vi "VI Anlagenuebersicht PNS.vi"() -> (3 "XML-String":string)   [LabVIEW 2015, in "Anlagenuebersicht.lvlib"]
uses:
  VisBx Anzeige/Anlagenuebersicht.lvlib
  VisBx Anzeige/PNS Uebersicht.ctl
panel:
  # "PNS"
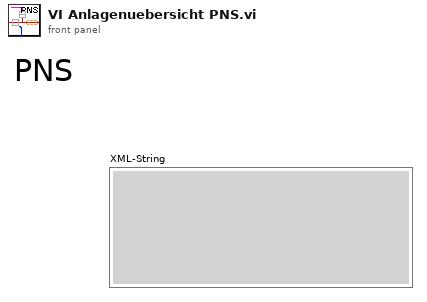
[diagram p1: front panel]
types:
  T1 = typedef "Anlagenuebersicht.lvlib/PNS Uebersicht.ctl" = cluster{"VFS 1 Y1":bool, "VFS 1 Y2":bool, "VFS 1 Y3":bool, "VFS 1 Y4":bool, "VFS 1 Y Reserve1":bool, "VFS 1 Y Reserve2":bool, "VFS 2 Y1":bool, "VFS 2 Y2":bool, "VFS 2 Y3":bool, "VFS 2 Y4":bool, "VFS 2 Y Reserve1":bool, "VFS 2 Y Reserve2":bool, "VFS 3 Y1":bool, "VFS 3 Y2":bool, "VFS 3 Y3":bool, "VFS 3 Y4":bool, "VFS 3 Y Reserve1":bool, "VFS 3 Y Reserve2":bool, "VFS 4 Y1":bool, "VFS 4 Y2":bool, "VFS 4 Y3":bool, "VFS 4 Y4":bool, "VFS 4 Y Reserve1":bool, "VFS 4 Y Reserve2":bool, "Zustand":enum16{"Stby/Pause/Eco", "Messen", "Spülen Filter", "Spülen Leitung", "Umgebungsluft", "0-Gas / Hintergrund", "Cal-Gas"}}
  T2 = enum16{"Stby/Pause/Eco", "Messen", "Spülen Filter", "Spülen Leitung", "Umgebungsluft", "0-Gas / Hintergrund", "Cal-Gas"}
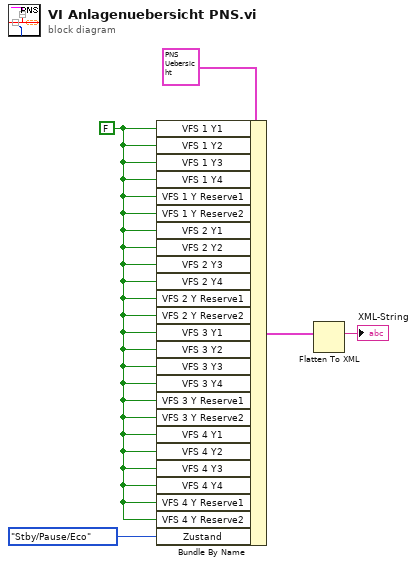
[diagram p0: block diagram]
diagram:
  w1 = FALSE ("-17S2")
  n1 = Bundle By Name(cluster=T1 {"VFS 1 Y1"=FALSE, "VFS 1 Y2"=FALSE, "VFS 1 Y3"=FALSE, "VFS 1 Y4"=FALSE, "VFS 1 Y Reserve1"=FALSE, "VFS 1 Y Reserve2"=FALSE, "VFS 2 Y1"=FALSE, "VFS 2 Y2"=FALSE, "VFS 2 Y3"=FALSE, "VFS 2 Y4"=FALSE, "VFS 2 Y Reserve1"=FALSE, "VFS 2 Y Reserve2"=FALSE, "VFS 3 Y1"=FALSE, "VFS 3 Y2"=FALSE, "VFS 3 Y3"=FALSE, "VFS 3 Y4"=FALSE, "VFS 3 Y Reserve1"=FALSE, "VFS 3 Y Reserve2"=FALSE, "VFS 4 Y1"=FALSE, "VFS 4 Y2"=FALSE, "VFS 4 Y3"=FALSE, "VFS 4 Y4"=FALSE, "VFS 4 Y Reserve1"=FALSE, "VFS 4 Y Reserve2"=FALSE, "Zustand"=enum."Stby/Pause/Eco"} ("Messwerte"), "VFS 1 Y1"=w1, "VFS 1 Y2"=w1, "VFS 1 Y3"=w1, "VFS 1 Y4"=w1, "VFS 1 Y Reserve1"=w1, "VFS 1 Y Reserve2"=w1, "VFS 2 Y1"=w1, "VFS 2 Y2"=w1, "VFS 2 Y3"=w1, "VFS 2 Y4"=w1, "VFS 2 Y Reserve1"=w1, "VFS 2 Y Reserve2"=w1, "VFS 3 Y1"=w1, "VFS 3 Y2"=w1, "VFS 3 Y3"=w1, "VFS 3 Y4"=w1, "VFS 3 Y Reserve1"=w1, "VFS 3 Y Reserve2"=w1, "VFS 4 Y1"=w1, "VFS 4 Y2"=w1, "VFS 4 Y3"=w1, "VFS 4 Y4"=w1, "VFS 4 Y Reserve1"=w1, "VFS 4 Y Reserve2"=w1, "Zustand"=T2."Stby/Pause/Eco") -> (w5:T1)
  n2 = Flatten To XML(anything=w5) -> (xml string=→"XML-String":string)
